vi "testDataPass_v2,1_vi0.vi"() -> ()   [LabVIEW 2014]
uses:
  testDataPass_v2,0_global1.vi
panel:
  out "error out 3":errorcluster
  out "error out 2":errorcluster
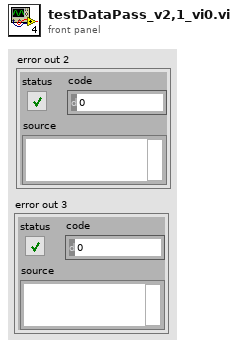
[diagram p1: front panel]
types:
  T1 = enum32{"Invalid", "Standard", "Closed", "Hidden", "Minimized", "Maximized"}
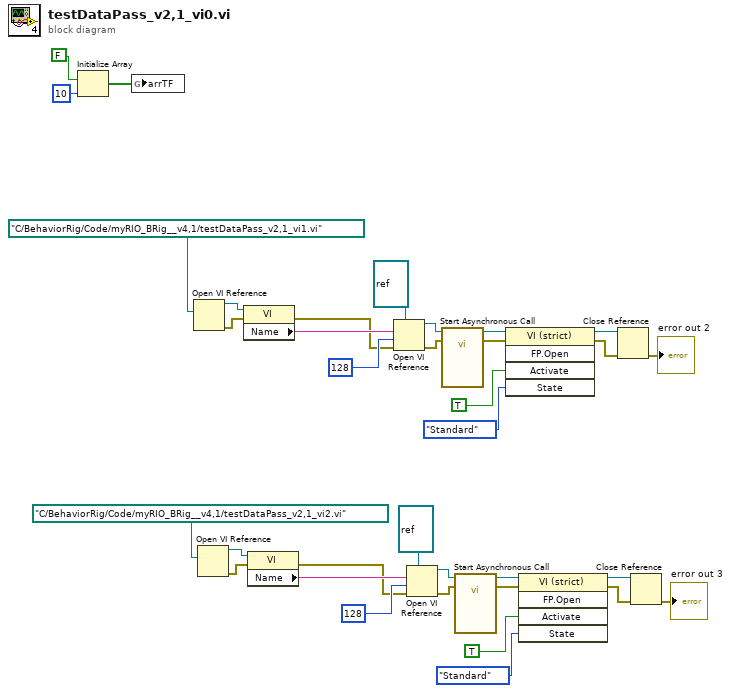
[diagram p0: block diagram]
diagram:
  n1 = Initialize Array(FALSE, 10 ("dimension size")) -> (w35:bool[])
  n2 = global write "testDataPass_v2,0_global1.vi" "arrTF"(w35) -> ()
  n3 = Open VI Reference(vi path=path "C:/BehaviorRig/Code/myRIO_BRig__v4,1/testDataPass_v2,1_vi1.vi") -> (vi reference=w26:refnum<vi>, error out=w27:errorcluster)  [unwired: 5 in]
  n4 = Open VI Reference(vi path=path "C:/BehaviorRig/Code/myRIO_BRig__v4,1/testDataPass_v2,1_vi2.vi") -> (vi reference=w15:refnum<vi>, error out=w16:errorcluster)  [unwired: 5 in]
  n5 = property class="VI"(reference=w26, error in=w27) -> (error out=w17:errorcluster, "Name"=w25:string)  [unwired: 1 out]
  n6 = property class="VI"(reference=w15, error in=w16) -> (error out=w2:errorcluster, "Name"=w3:string)  [unwired: 1 out]
  n7 = Open VI Reference(type specifier VI Refnum (for type only)=refnum<vi> refnum, vi path=w25, options=128, error in (no error)=w17) -> (vi reference=w31:refnum<vi>, error out=w30:errorcluster)  [unwired: 2 in]
  n8 = Open VI Reference(type specifier VI Refnum (for type only)=refnum<vi> refnum, vi path=w3, options=128, error in (no error)=w2) -> (vi reference=w12:refnum<vi>, error out=w11:errorcluster)  [unwired: 2 in]
  n9 = call-by-ref "Start Asynchronous Call"(reference=w31, error in=w30) -> (reference out=w23:refnum<vi>, error out=w22:errorcluster)  [unwired: 12 in]
  n10 = call-by-ref "Start Asynchronous Call"(reference=w12, error in=w11) -> (reference out=w9:refnum<vi>, error out=w8:errorcluster)  [unwired: 12 in]
  n11 = invoke class="VI (strict)" method="FP.Open"(reference=w23, error in=w22, "Activate"=TRUE ("Activate?"), "State"=T1."Standard") -> (reference out=w19:refnum<vi>, error out=w18:errorcluster)  [unwired: 1 in, 3 out]
  n12 = invoke class="VI (strict)" method="FP.Open"(reference=w9, error in=w8, "Activate"=TRUE ("Activate?"), "State"=T1."Standard") -> (reference out=w5:refnum<vi>, error out=w4:errorcluster)  [unwired: 1 in, 3 out]
  n13 = Close Reference(reference=w19, error in (no error)=w18) -> (error out=→"error out 2":errorcluster)
  n14 = Close Reference(reference=w5, error in (no error)=w4) -> (error out=→"error out 3":errorcluster)
